vi "Scan time Input.vi"(11 "In":u32=30) -> (3 "out":u32)   [LabVIEW 2011]
uses:
  <vilib>/Utility/miscctls.llb/LVSelectionTypeDef.ctl
panel:
  in  "cancel":bool
  in  "ok":bool
  in  "Scan Time":u32=10 caption="请输入数值：" min=1 max=10000 step=1
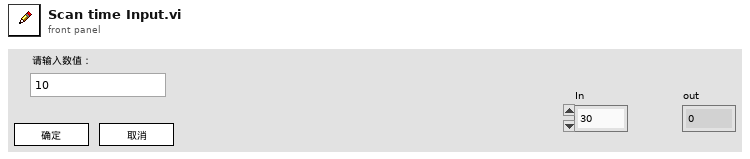
[diagram p1: front panel]
types:
  T1 = typedef "LVSelectionTypeDef.ctl" = cluster{"Selection Start":u32, "Selection End":u32}
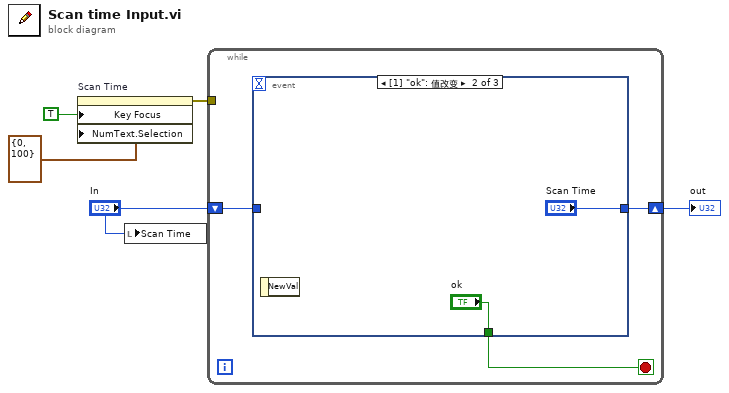
[diagram p0: block diagram]
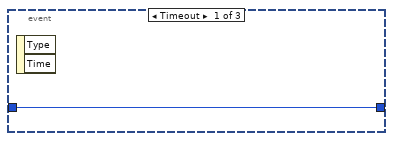
[diagram p2: hidden frame]
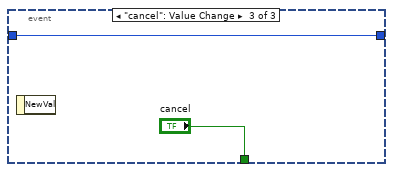
[diagram p3: hidden frame]
diagram:
  n1 = property on="Scan Time" class="DigNum (严格)"("Key Focus"=TRUE ("键选中"), "NumText.Selection"=T1 {"Selection Start"=0, "Selection End"=100} ("数值文本.选择")) -> (error out=w4:errorcluster)  [unwired: 2 in, 1 out]
  n2 = local write "Scan Time"("In") -> ()
  n3 = while {
    shift-right: [w7] -> w5
    shift-left: "In" -> [w8]
    tunnel: w4 -> [_]
    stop <- w6 stop-if-true
    n4 = event shown="[1] \"ok\": 值改变" {
      selector: _ -> [_ _ _]
      dyn-events: _ -> [_ _ _]
      timeout: _ -> [_ _ _]
      tunnel: w8 -> [w9 _ w12]
      tunnel: [w9 "Scan Time" w12] -> w7
      tunnel: [_ "ok" "cancel"] -> w6
      event Timeout {
        n5 = event-data() -> ()  [unwired: 1 in, 2 out]
      }
      event "ok": Value Change {
        n6 = event-data() -> ()  [unwired: 1 in, 1 out]
      }
      event "cancel": Value Change {
        n7 = event-data() -> ()  [unwired: 1 in, 1 out]
      }
    }
  }
  "out" <- w5
